vi "Actuate HW.vi"(8 "error in (no error)":errorcluster, 11 "DAQmx Switch in":refnum<class "DAQmx Switch.lvclass">) -> (0 "error out":errorcluster, 3 "DAQmx Switch out":refnum<class "DAQmx Switch.lvclass">)   [LabVIEW 2020, in "DAQmx Switch.lvclass"]
uses:
  DAQmx Switch.lvclass
  C:/Users/jharw/Documents/1 Folder to Rule them All/UMD/Inflation-Apparatus/src/Hardware/Actuators/Switches/Switch.lvclass
  Switch.lvclass/Switch.ctl
  DAQmx Switch.lvclass/DAQmx Switch.ctl
  <vilib>/DAQmx/write.llb/DAQmx Write (Digital Bool 1Line 1Point).vi
  <vilib>/DAQmx/miscellaneous.llb/DAQmx Fill In Error Info.vi
  Switch.lvclass
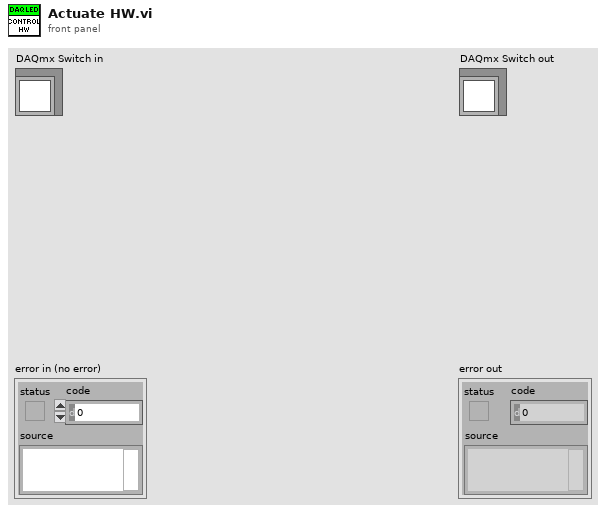
[diagram p1: front panel]
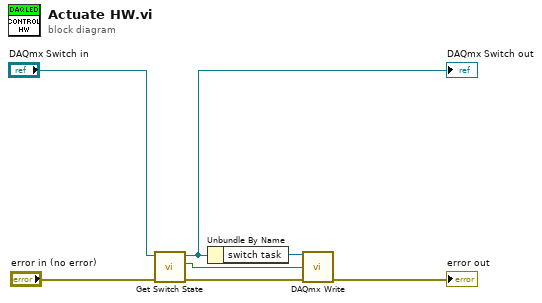
[diagram p0: block diagram]
diagram:
  n1 = call "Get Switch State.vi"("error in (no error)"="error in (no error)", "Switch in"="DAQmx Switch in") -> ("error out"=w5:errorcluster, "switch state"=w2:bool, "Switch out"=w1:refnum<class "DAQmx Switch.lvclass">)  [unwired: 7 in]
  "DAQmx Switch out" <- w1
  n2 = Unbundle By Name(w1) -> ("switch task"=w3:refnum<k21>)
  n3 = call-poly <vilib>:"DAQmx Write.vi"("task/channels in"=w3, "data"=w2, "error in"=w5) -> ("error out"=→"error out":errorcluster)  [unwired: 10 in, 2 out]
